vi "Input FIFO Status.vi"(7 "error in":errorcluster, 8 "input.Reset":bool, 9 "input.FIFO Size":u32, 10 "FPGA VI Reference":refnum<k20>) -> (0 "error out":errorcluster, 1 "input.Ever Timed Out?":bool caption="Ever Timed Out?", 2 "input.Throughput (B/s)":dbl caption="Throughput (B/s)" format="%#.3p", 3 "input.FPGA FIFO Status":cluster{u32, u32}(slide) caption="FPGA FIFO Status" scale=0.0..32000.0 scale format="%#.1p")   [LabVIEW 2013]
doc: "This SubVI Monitors the Status of the Host to Target DMA FPGA FIFO and returns the actual achieved throughput."
uses:
  <vilib>/rvi/interface/nirviReadWriteControl/nirviReadWriteControl.xnode
  NiFpgaLv.dll
  <vilib>/Utility/error.llb/Error Cluster From Error Code.vi
  <vilib>/rvi/interface/Simulation/niFpgaSimulationCallBeginRW.vi
  <vilib>/rvi/errors/niLvFpgaAdjustHostInterfaceError.vi
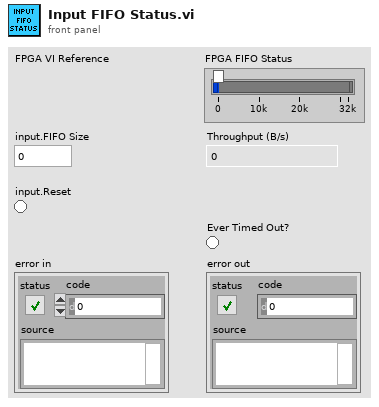
[diagram p1: front panel]
types:
  T1 = cluster{"Iterations":u64, "Number of Elements Written":u64}
  T2 = cluster{"Current Amount Used":u32, "Maximum Amount Used":u32}
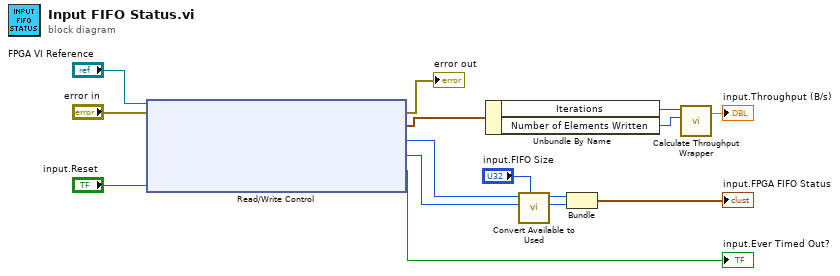
[diagram p0: block diagram]
diagram:
  n1 = xnode "Read/Write Control"("FPGA VI Reference In"="FPGA VI Reference", "error in"="error in", "input.Reset"="input.Reset") -> ("error out"=→"error out":errorcluster, "input.FIFO Transfer Status"=w1:T1, "input.Number of Elements to Write"=w15:u32, "input.Minimum Number of Elements to Write"=w14:u32, "input.Ever Timed Out?"=→"input.Ever Timed Out?":bool)  [unwired: 1 out]
  n2 = Unbundle By Name(w1) -> ("Iterations"=w3:u64, "Number of Elements Written"=w2:u64)
  n3 = call "Convert Available to Used.vi"("Size"="input.FIFO Size", "Minimum Amount Available"=w14, "Current Amount Available"=w15) -> ("Maximum Amount Used"=w12:u32, "Current Amount Used"=w13:u32)  [unwired: 5 in]
  n4 = Bundle("Current Amount Used"=w13, "Maximum Amount Used"=w12) -> (→"input.FPGA FIFO Status":T2)  [unwired: 1 in]
  n5 = call "Calculate Throughput Wrapper.vi"("transfers"=w2, "iterations"=w3) -> ("throughput (B/s)"=→"input.Throughput (B/s)":dbl)  [unwired: 3 in]
